vi "test_program_vi.vi"(0 "instrument handle":refnum<k15>, 1 "t_check":dbl, 3 "关断电压":dbl, 4 "中断电压":dbl, 5 "工作频率":dbl caption="Freq", 6 "t_on":dbl, 8 "t_off":dbl, 9 "直流偏置":dbl caption="Dcv", 10 "t_gap":dbl, 11 "工作电压":dbl caption="Acv", 12 "error in (no error)":errorcluster {"code" format="%.0x"}) -> (14 "instrument handle out":refnum<k15>, 15 "error out":errorcluster {"code" format="%.0x"})   [LabVIEW 2020]
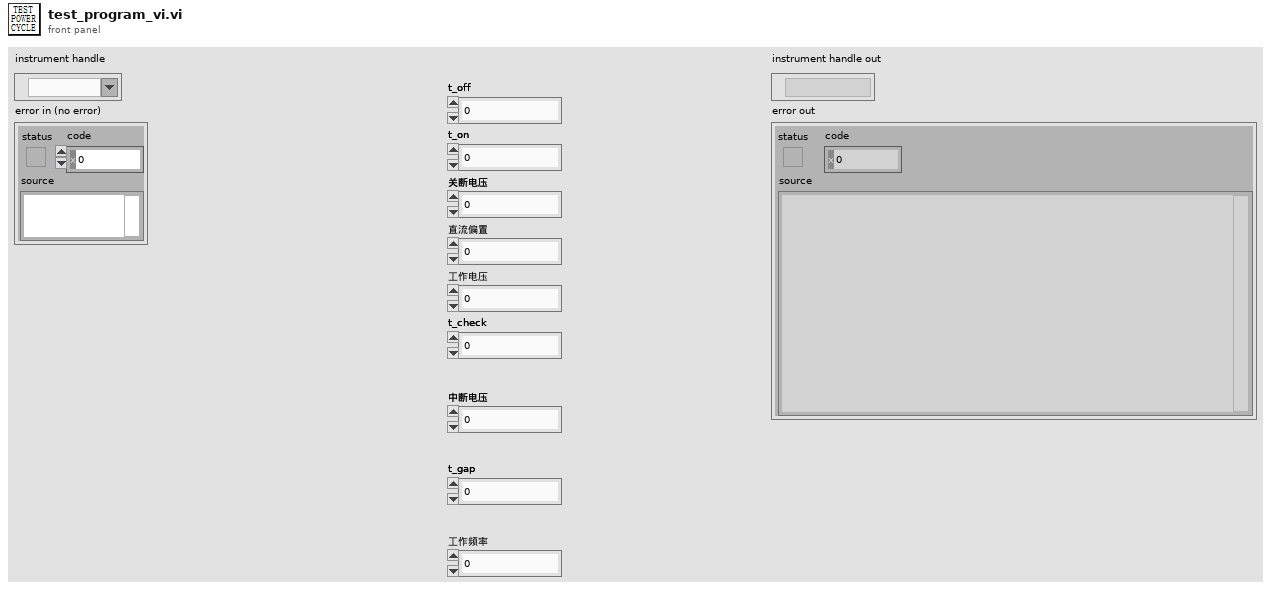
[diagram p1: front panel]
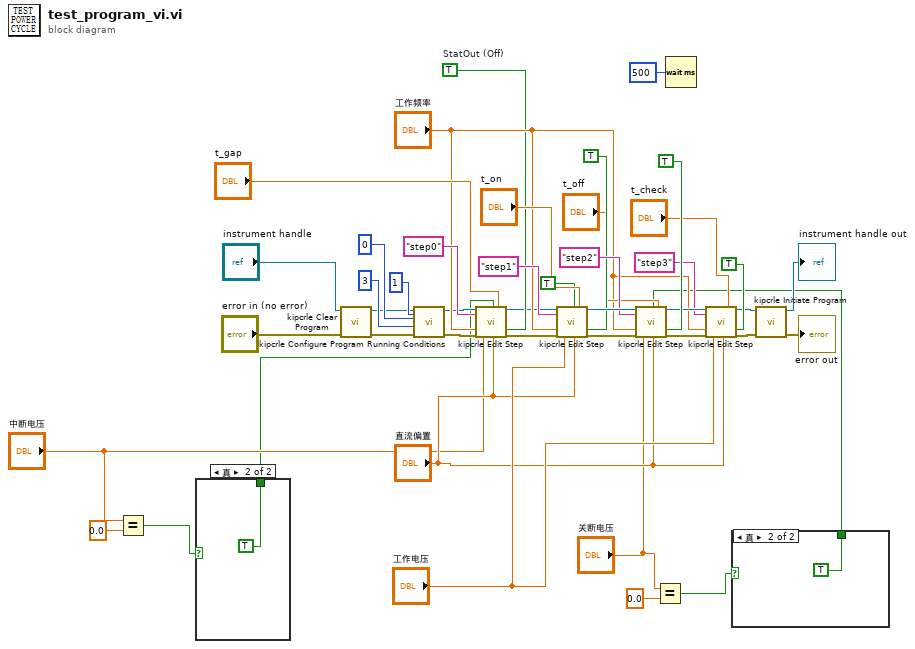
[diagram p0: block diagram]
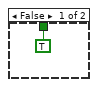
[diagram p2: hidden frame]
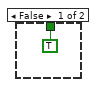
[diagram p3: hidden frame]
diagram:
  w17 = TRUE  # StatOut (Off)
  n1 = Equal?(x="中断电压", y=0.0) -> (x = y?=w7:bool)
  n2 = case shown="真" w7 {
    tunnel: [TRUE ("OutputEnabled (Off)") TRUE ("OutputEnabled (Off)")] -> w6
    frame False {
    }
    frame True {
    }
  }
  n3 = call <instrlib>:"kipcrle Clear Program.vi"("error in (no error)"="error in (no error)", "instrument handle"="instrument handle") -> ("error out"=w36:errorcluster, "instrument handle out"=w37:refnum<k15>)  [unwired: 8 in]
  n4 = call <instrlib>:"kipcrle Configure Program Running Conditions.vi"("Loop"=1, "error in (no error)"=w36, "EndPosition"=3, "StartPosition"=0, "instrument handle"=w37) -> ("error out"=w13:errorcluster, "instrument handle out"=w16:refnum<k15>)  [unwired: 5 in]
  n5 = call <instrlib>:"kipcrle Edit Step.vi"("instrument handle"=w16, "Step"="step0", "Freq"="工作频率", "error in (no error)"=w13, "Acv"="中断电压", "OutputEnabled (Off)"=w6, "Dcv"="直流偏置", "Time"="t_gap", "StatOut (Off)"=w17) -> ("instrument handle out"=w15:refnum<k15>, "error out"=w12:errorcluster)  [unwired: 9 in]
  n6 = call <instrlib>:"kipcrle Edit Step.vi"("instrument handle"=w15, "Step"="step1", "Freq"="工作频率", "error in (no error)"=w12, "Acv"="工作电压", "OutputEnabled (Off)"=TRUE, "Dcv"="直流偏置", "Time"="t_on", "StatOut (Off)"=TRUE) -> ("instrument handle out"=w34:refnum<k15>, "error out"=w33:errorcluster)  [unwired: 9 in]
  n7 = Equal?(x="关断电压", y=0.0) -> (x = y?=w1:bool)
  n8 = Wait (ms)(milliseconds to wait=u32 500 ("等待时间（毫秒）")) -> ()  [unwired: 1 out]
  n9 = case shown="真" w1 {
    tunnel: [TRUE ("OutputEnabled (Off)") TRUE ("OutputEnabled (Off)")] -> w2
    frame False {
    }
    frame True {
    }
  }
  n10 = call <instrlib>:"kipcrle Edit Step.vi"("instrument handle"=w34, "Step"="step2", "Freq"="工作频率", "error in (no error)"=w33, "Acv"="关断电压", "OutputEnabled (Off)"=w2, "Dcv"="直流偏置", "Time"="t_off", "StatOut (Off)"=TRUE) -> ("instrument handle out"=w29:refnum<k15>, "error out"=w28:errorcluster)  [unwired: 9 in]
  n11 = call <instrlib>:"kipcrle Edit Step.vi"("instrument handle"=w29, "Step"="step3", "Freq"="工作频率", "error in (no error)"=w28, "Acv"="工作电压", "Dcv"="直流偏置", "Time"="t_check", "StatOut (Off)"=TRUE) -> ("instrument handle out"=w14:refnum<k15>, "error out"=w11:errorcluster)  [unwired: 10 in]
  n12 = call <instrlib>:"kipcrle Initiate Program.vi"("error in (no error)"=w11, "instrument handle"=w14) -> ("error out"=→"error out":errorcluster, "instrument handle out"=→"instrument handle out":refnum<k15>)  [unwired: 8 in]
